vi "lab.vi"() -> ()   [LabVIEW 2020]
panel:
  in  "min(V) 2":dbl
  in  "max(V) 2":dbl
  in  "step(V) 2":dbl
  out "array":dbl[](array[numeric])
  out "I":dbl[](array[numeric])
  out "V":dbl[](array[numeric])
  in  "step(V)":dbl
  in  "max(V)":dbl
  in  "min(V)":dbl
  out "R":dbl
  out "XY Graph":cluster{"X":dbl, "Y":dbl}[](graph)
  out "Measurements":dbl
  in  "Auto Zero (0: Enable)":u32(ring) items=["Enable", "Disable", "Once"]
  in  "Auto Range (T: Enable)":bool=TRUE
  in  "Function (0: Voltage DC)":i32(ring) items=[" Voltage DC", "Voltage AC", "Current DC", "Current AC", "Resistance", "4-wire Resistance", "Diode", "Capacitance", "Temperature", "Continuity", "Frequency", "Period", "Voltage Ratio", "Digitize Voltage", "Digitize Current"]
  in  "Manual Range (0)":dbl
  in  "VISA resource name 2":refnum<visa-resource-name>
  out "Measured Current":sgl
  out "Measured Voltage":sgl
  in  "Output Current":dbl=1.0
  in  "Supply Voltage":dbl
  in  "Output State":u16(ring) items=["OFF", "ON"]
  in  "Channel Control":u16(ring)=1 items=["N/A", "Channel 1", "Channel 2", "Channel 3"]
  out "VISA resource name out":refnum<visa-resource-name>
  in  "Reset? (T: Yes)":bool=TRUE
  in  "VISA resource name":refnum<visa-resource-name>
  # "电压源 2231A-30-A"
  # "万用表 DMM6500"
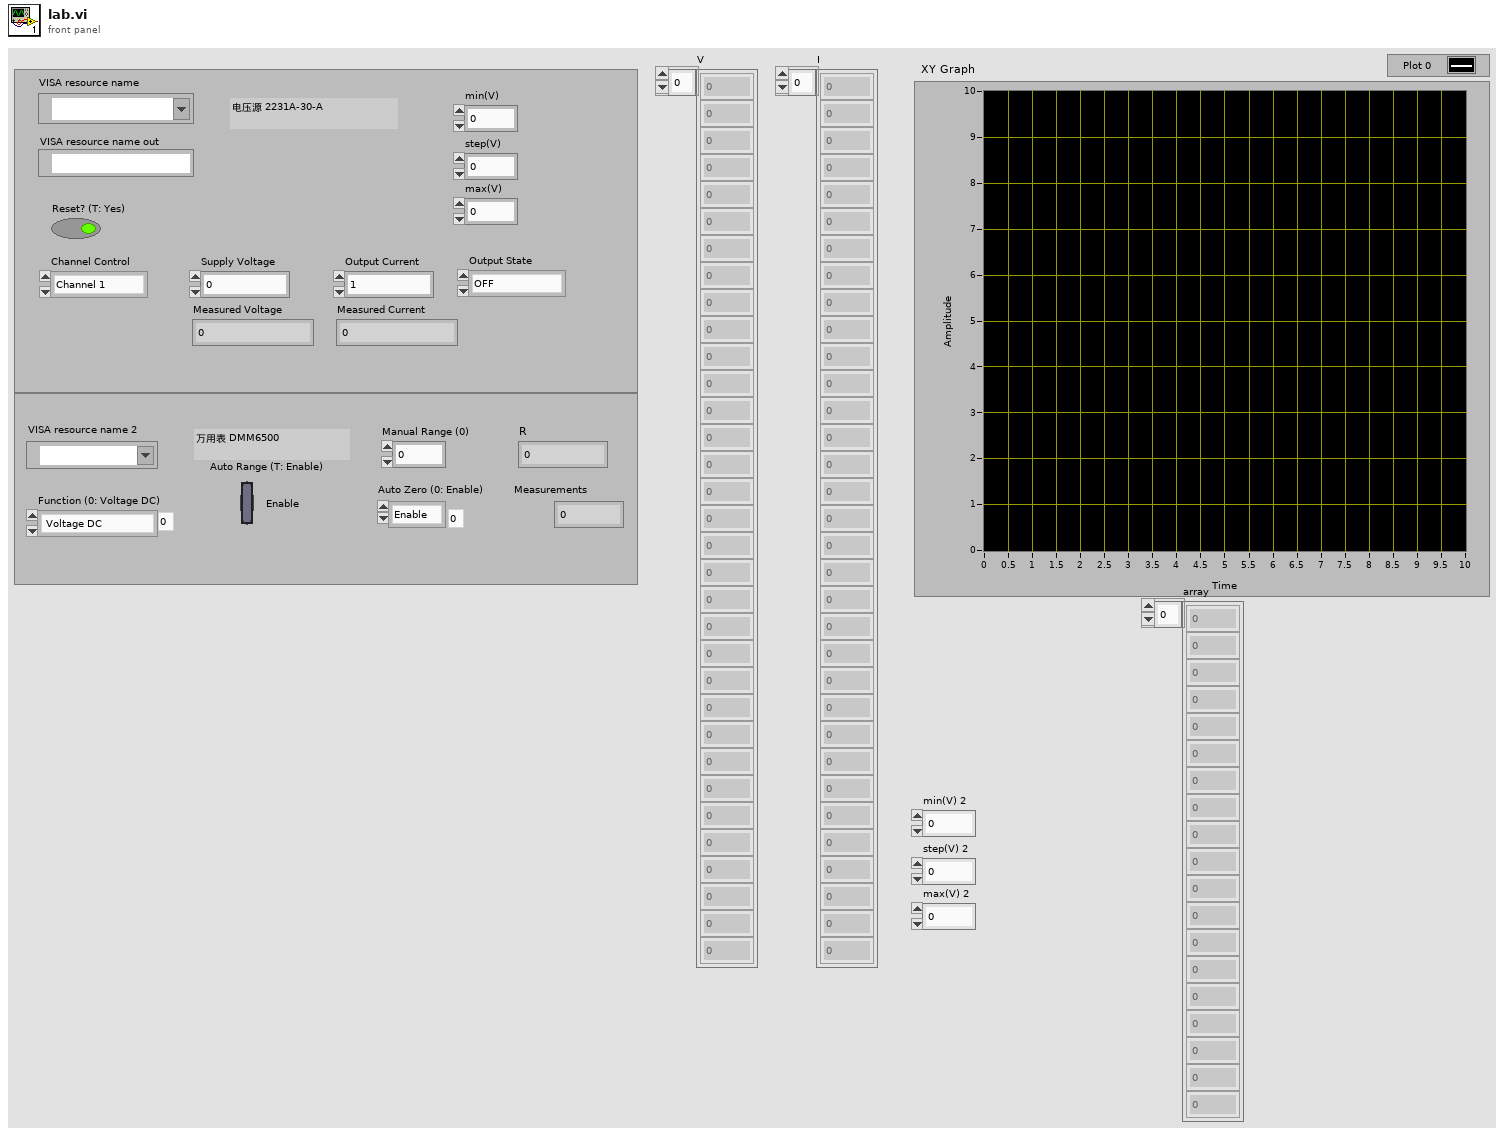
[diagram p1: front panel]
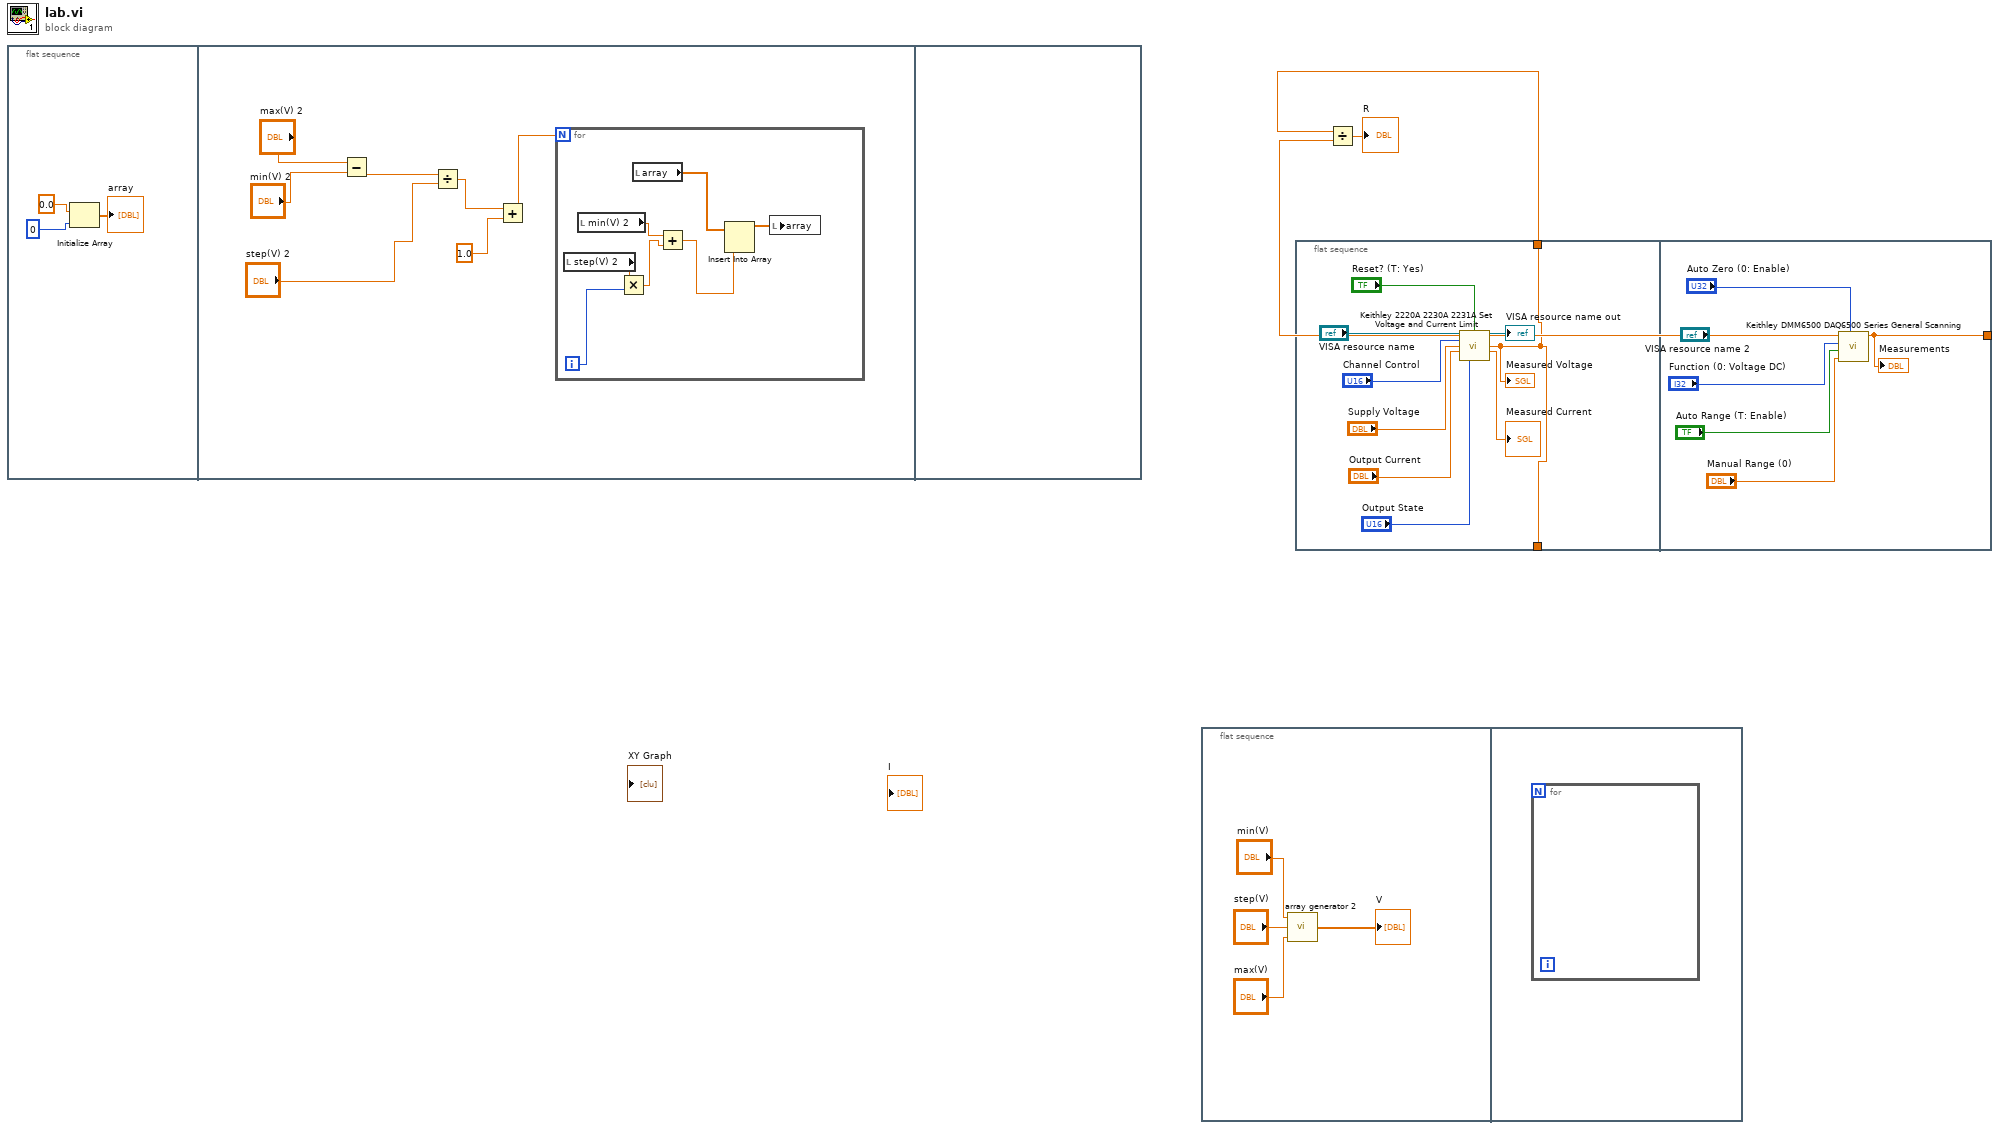
[diagram p0: block diagram]
diagram:
  n1 = flat-sequence {
    frame #0 {
      n2 = Initialize Array(0.0 ("element"), 0 ("dimension size")) -> (→"array":dbl[])
    }
    frame #1 {
      n3 = Subtract(x="max(V) 2", y="min(V) 2") -> (x-y=w11:dbl)
      n4 = Divide(x=w11, y="step(V) 2") -> (x/y=w9:dbl)
      n5 = Add(x=w9, y=1.0) -> (x+y=w7:dbl)
      n6 = for {
        N: w7 -> [_]
        i -> [w18]
        n7 = local read "step(V) 2"() -> (w17:dbl)
        n8 = local read "min(V) 2"() -> (w19:dbl)
        n9 = Multiply(x=w17, y=w18) -> (x*y=w16:dbl)
        n10 = local read "array"() -> (w20:dbl[])
        n11 = Add(x=w19, y=w16) -> (x+y=w14:dbl)
        n12 = Insert Into Array(array=w20, new element=w14) -> (w15:dbl[])  [unwired: 1 in]
        n13 = local write "array"(w15) -> ()
      }
    }
    frame #2 {
    }
  }
  n14 = flat-sequence {
    frame #0 {
      n15 = call "array generator 2.vi"("max(V)"="max(V)", "step(V)"="step(V)", "min(V)"="min(V)") -> ("array"=→"V":dbl[])
    }
    frame #1 {
      n16 = for {
      }
    }
  }
  n17 = flat-sequence {
    tunnel: [w25] -> w2
    tunnel: [w25] -> _
    tunnel: [w34] -> w1
    frame #0 {
      n18 = call "Keithley 2220A 2230A 2231A Set Voltage and Current Limit.vi"("VISA resource name"="VISA resource name", "Reset? (T: Yes)"="Reset? (T: Yes)", "Channel Control"="Channel Control", "Supply Voltage"="Supply Voltage", "Output Current"="Output Current", "Output State"="Output State") -> ("VISA resource name out"=→"VISA resource name out":refnum<visa-resource-name>, "Measured Voltage"=w25:sgl, "Measured Current"=→"Measured Current":sgl)  [unwired: 6 in, 1 out]
      "Measured Voltage" <- w25
    }
    frame #1 {
      n19 = call "Keithley DMM6500 DAQ6500 Series General Scanning.vi"("Auto Zero (0: Enable)"="Auto Zero (0: Enable)", "Manual Range (0)"="Manual Range (0)", "Auto Range (T: Enable)"="Auto Range (T: Enable)", "Function (0: Voltage DC)"="Function (0: Voltage DC)", "VISA resource name"="VISA resource name 2") -> ("Measurements"=w34:dbl)  [unwired: 6 in]
      "Measurements" <- w34
    }
  }
  n20 = Divide(x=w2, y=w1) -> (x/y=→"R":dbl)
